vi "goToStandby.vi"(8 "error in (no error)":errorcluster, 10 "model in":refnum<class "IModel.lvclass">, 11 "DisabledState in":refnum<class "DisabledState.lvclass">) -> (0 "error out":errorcluster, 2 "model out":refnum<class "IModel.lvclass">, 3 "DisabledState out":refnum<class "DisabledState.lvclass">)   [LabVIEW 2015, in "States.lvlib" / "DisabledState.lvclass"]
uses:
  DisabledState.lvclass
  IModel/IModel.lvclass
  Typedefs/StateValue.ctl
  ComponentTemplateCore/ComponentModel/ComponentModel/Typedefs/ComponentStateValues.ctl
  ComponentTemplateCore/ComponentModel/ComponentModel/InternalSignals/restart.vi
  Typedefs/EXATypedefs.lvlib
  ComponentTemplateCore/ComponentModel/ComponentModel/InternalSignals/InternalSignalsGlobals.lvlib
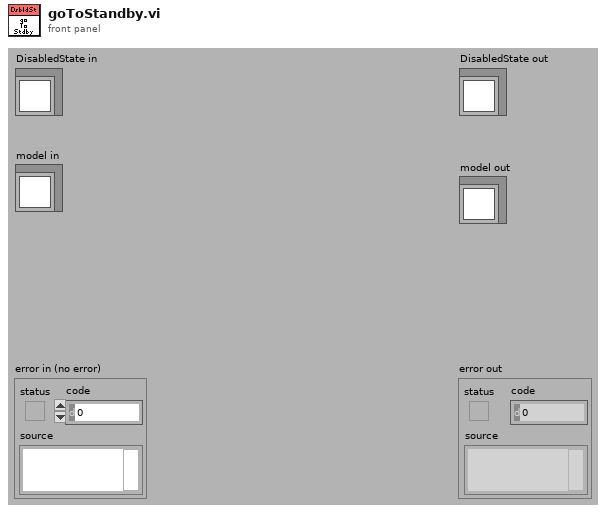
[diagram p1: front panel]
types:
  T1 = typedef "componentStateValues.ctl" = enum16{"Off", "Standby", "Enabled", "Disabled", "Fault"}
  T2 = typedef "EXATypedefs.lvlib/StateValue.ctl" = enum16{"DisabledState", "EnabledState", "FaultState", "OffState", "StandbyState"}
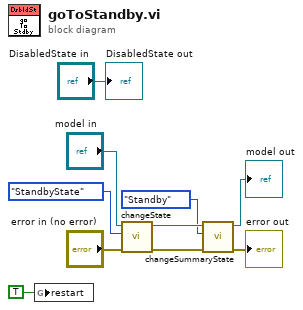
[diagram p0: block diagram]
diagram:
  n1 = global write "restart.vi" "restart"(TRUE ("restart")) -> ()
  n2 = call-dynamic "changeState.vi"("error in (no error)"="error in (no error)", "newState"=StateValue."StandbyState" ("StateValue"), "IModel in"="model in") -> ("error out"=w6:errorcluster, "IModel out"=w5:refnum<class "IModel.lvclass">)  [unwired: 7 in]
  n3 = call-dynamic "changeSummaryState.vi"("error in (no error)"=w6, "newSummaryState"=componentStateValues."Standby" ("componentStateValues"), "IModel in"=w5) -> ("error out"=→"error out":errorcluster, "IModel out"=→"model out":refnum<class "IModel.lvclass">)  [unwired: 7 in]
  "DisabledState out" <- "DisabledState in"
